vi "Evaluate Scope.vi"(10 "call chain":string[](array[string]), 11 "basic scope":refnum<class "Basic.lvclass">) -> (2 "matches":bool[](array[boolean]), 3 "dup basic scope":refnum<class "Basic.lvclass">)   [LabVIEW 2018, in "GLog.lvlib" / "Basic.lvclass"]
uses:
  Basic.lvclass
  Basic.lvclass/Basic.ctl
panel:
  # "Connector Pane"
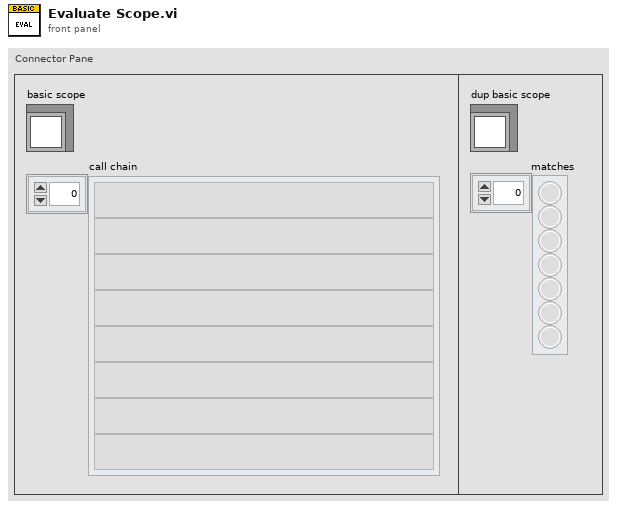
[diagram p1: front panel]
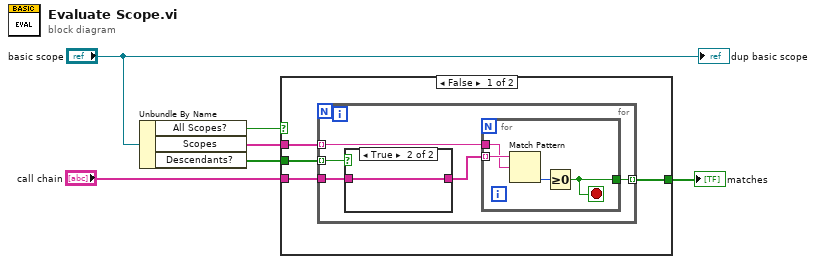
[diagram p0: block diagram]
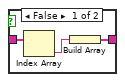
[diagram p2: hidden frame]
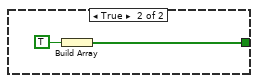
[diagram p3: hidden frame]
diagram:
  n1 = Unbundle By Name("basic scope") -> ("All Scopes?"=w2:bool, "Scopes"=w3:string[], "Descendants?"=w1:bool[])
  n2 = case shown="False" w2 {
    tunnel: "call chain" -> [w10 _]
    tunnel: [w9 w24] -> w4
    tunnel: w3 -> [w8 _]
    tunnel: w1 -> [w7 _]
    frame False {
      n3 = for {
        tunnel: w10 -> [w15]
        tunnel: w8 -> [w14] mode=indexing
        tunnel: [w13] -> w9 mode=indexing
        tunnel: w7 -> [w11] mode=indexing
        n4 = case shown="True" w11 {
          tunnel: w15 -> [w18 w19]
          tunnel: [w16 w19] -> w12
          frame False {
            n5 = Index Array(array=w18) -> (element=w17:string)  [unwired: 1 in]
            n6 = Build Array(w17) -> (w16:string[])
          }
          frame True {
          }
        }
        n7 = for {
          tunnel: w12 -> [w23] mode=indexing
          tunnel: w14 -> [w22]
          tunnel: [w20] -> w13
          stop <- w20 stop-if-true
          n8 = Match Pattern(string=w23, regular expression=w22) -> (offset past match=w21:i32)  [unwired: 1 in, 3 out]
          n9 = Greater Or Equal To 0?(x=w21) -> (x >= 0?=w20:bool)
        }
      }
    }
    frame True {
      n10 = Build Array(TRUE) -> (w24:bool[])
    }
  }
  "matches" <- w4
  "dup basic scope" <- "basic scope"
